vi "move_to.vi"(4 "error in (no error)":errorcluster, 6 "Request data":variant, 7 "Python session in":refnum<k35>) -> (0 "error out":errorcluster, 2 "Response data":variant, 3 "Python session out":refnum<k35>)   [LabVIEW 2018]
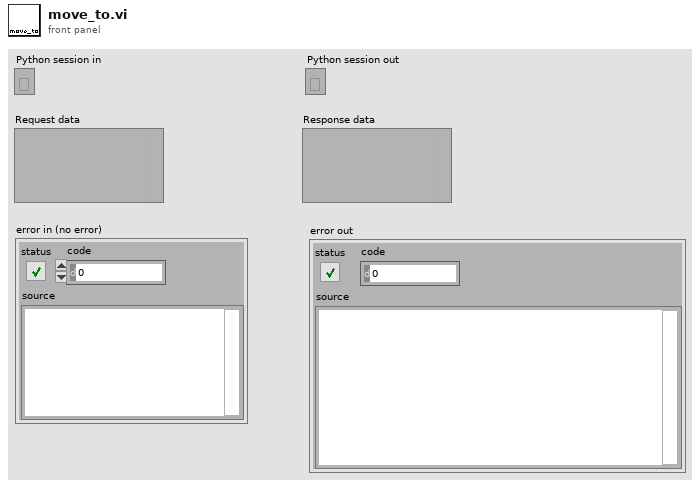
[diagram p1: front panel]
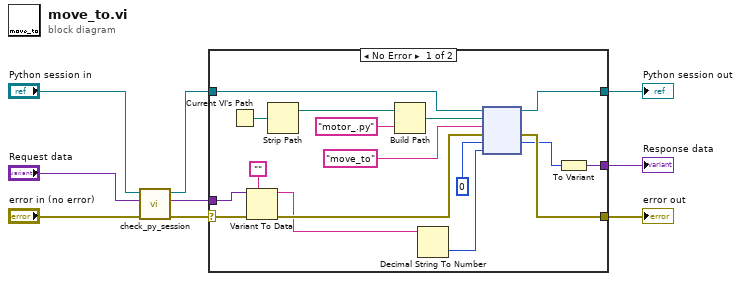
[diagram p0: block diagram]
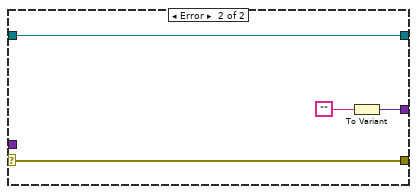
[diagram p2: hidden frame]
diagram:
  n1 = call "check_py_session.vi"("error in"="error in (no error)", "Request data"="Request data", "Python session in"="Python session in") -> ("error out"=w3:errorcluster, "Response data"=w4:variant, "Python session out"=w5:refnum<k35>)  [unwired: 2 in]
  n2 = case shown="No Error" w3 {
    selector: w3 -> [w18 w30]
    tunnel: w5 -> [w26 w29]
    tunnel: [w20 w29] -> w9
    tunnel: w4 -> [w19 _]
    tunnel: [w16 w30] -> w2
    tunnel: [w15 w27] -> w1
    frame No Error {
      n3 = Current VI's Path() -> (path=w22:path)
      n4 = Variant To Data(error in=w18, type="", Variant=w19) -> (data=w11:string, error out=w17:errorcluster)
      n5 = Strip Path(path=w22) -> (stripped path=w21:path)  [unwired: 1 out]
      n6 = Build Path(base path=w21, name or relative path="motor_.py") -> (appended path=w24:path)
      n7 = Decimal String To Number(string=w11) -> (number=w10:i32)  [unwired: 2 in, 1 out]
      n8 = node(w26, w24, "move_to" ("function name"), w17, 0, w10) -> (w20:refnum<k35>, w16:errorcluster, w14:i32)  [unwired: 1 in, 2 out]
      n9 = To Variant(anything=w14) -> (Variant=w15:variant)
    }
    frame Error {
      n10 = To Variant(anything="") -> (Variant=w27:variant)
    }
  }
  "error out" <- w2
  "Python session out" <- w9
  "Response data" <- w1
